vi "Average_Reactor_Coolant_Temperature.vi"(8 "error in (no error)":errorcluster, 11 "AverageReactorCoolantTemperature.lvclass":refnum<class "AverageReactorCoolantTemperature.lvclass">) -> (0 "error out":errorcluster, 3 "AverageReactorCoolantTemperature.lvclass 2":refnum<class "AverageReactorCoolantTemperature.lvclass">)   [LabVIEW 2022 SP3, in "AverageReactorCoolantTemperature.lvclass"]
uses:
  AverageReactorCoolantTemperature.lvclass
  AverageReactorCoolantTemperature.lvclass/AverageReactorCoolantTemperature.ctl
panel:
  out "ACT 2ND MAX LIM":dbl
  out "ACT D-Comp":dbl
  out "ACT 2nd Ctrl":dbl
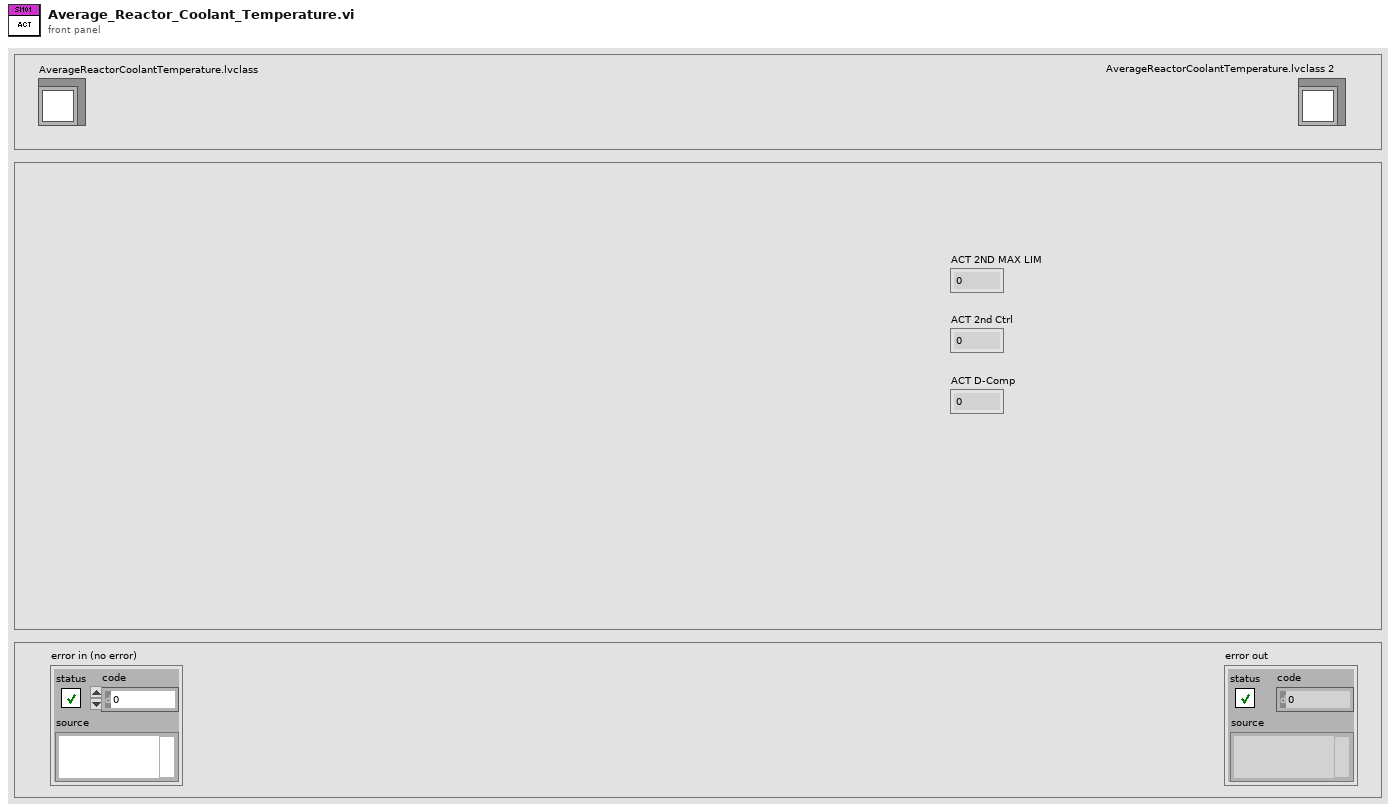
[diagram p1: front panel]
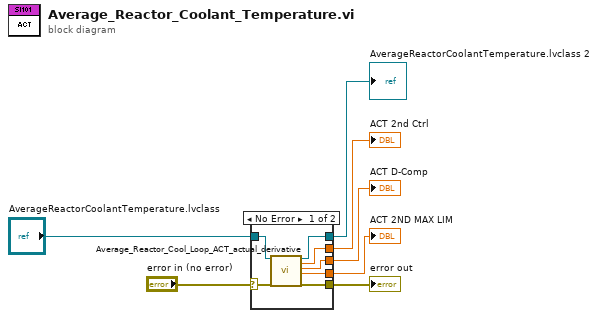
[diagram p0: block diagram]
diagram:
  n1 = case shown="No Error" "error in (no error)" {
    selector: "error in (no error)" -> [w11 w16]
    tunnel: [w13 w16] -> w6
    tunnel: [w14 w15] -> w1
    tunnel: "AverageReactorCoolantTemperature.lvclass" -> [w12 w15]
    tunnel: [w10 _] -> w5
    tunnel: [w9 _] -> w4
    tunnel: [w8 _] -> w3
    frame No Error {
      n2 = call "Average_Reactor_Cool_Loop_ACT_actual_derivative.vi"("SI101_AverageReactorCoolantTemperature.lvclass"=w12, "error in (no error)"=w11) -> ("SI101_AverageReactorCoolantTemperature.lvclass out"=w14:refnum<class "AverageReactorCoolantTemperature.lvclass">, "ACT 2nd Ctrl"=w10:dbl, "ACT D-Comp"=w9:dbl, "ACT 2ND MAX LIM"=w8:dbl, "error IO"=w13:errorcluster)  [unwired: 13 in]
    }
    frame Error {
    }
  }
  "error out" <- w6
  "ACT 2nd Ctrl" <- w5
  "ACT D-Comp" <- w4
  "ACT 2ND MAX LIM" <- w3
  "AverageReactorCoolantTemperature.lvclass 2" <- w1
